vi "MGI Bezier Find k.vi"(1 "y":sgl format="%.2f", 2 "first k":i32=1, 3 "Bezier Control Points[]":sgl[](array[numeric]) format="%.2f") -> (0 "correct k":i32)   [LabVIEW 2016]
doc: "Search the Bezier Control Points array for the block containing y. y is tested against y(first k + 3 + 4*n), where n = 0, 1, .... Return value is (first k + 4*n), suitable for input to Bezier Inverse.\n\nAuthored by David A. Moore\nsupport@mooregoodideas.com\nwww.mooregoodideas.com\n\nCopyright (c) 2010, Moore Good Ideas, Inc.\n\nAll rights reserved.\n\nRedistribution and use in source and binary forms, with or without modification, are permitted provided that the following conditions are met:\n\n * Redistributions of source code must retain the above copyright notice, this list of conditions and the following disclaimer.\n * Redistributions in binary form must reproduce the above copyright notice, this list of conditions and the following disclaimer in the documentation and/or other materials provided with the distribution.\n * Neither the name of Moore Good Ideas, Inc. nor the names of its contributors may be used to endorse or promote products derived from this software without specific prior written permission.\n\nTHIS SOFTWARE IS PROVIDED BY THE COPYRIGHT HOLDERS AND CONTRIBUTORS \"AS IS\" AND ANY EXPRESS OR IMPLIED WARRANTIES, INCLUDING, BUT NOT LIMITED TO, THE IMPLIED WARRANTIES OF MERCHANTABILITY AND FITNESS FOR A PARTICULAR PURPOSE ARE DISCLAIMED. IN NO EVENT SHALL THE COPYRIGHT OWNER OR CONTRIBUTORS BE LIABLE FOR ANY DIRECT, INDIRECT, INCIDENTAL, SPECIAL, EXEMPLARY, OR CONSEQUENTIAL DAMAGES (INCLUDING, BUT NOT LIMITED TO, PROCUREMENT OF SUBSTITUTE GOODS OR SERVICES; LOSS OF USE, DATA, OR PROFITS; OR BUSINESS INTERRUPTION) HOWEVER CAUSED AND ON ANY THEORY OF LIABILITY, WHETHER IN CONTRACT, STRICT LIABILITY, OR TORT (INCLUDING NEGLIGENCE OR OTHERWISE) ARISING IN ANY WAY OUT OF THE USE OF THIS SOFTWARE, EVEN IF ADVISED OF THE POSSIBILITY OF SUCH DAMAGE."
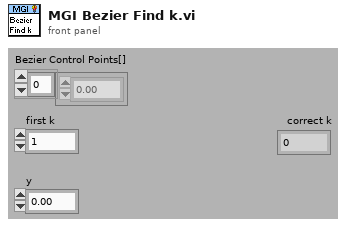
[diagram p1: front panel]
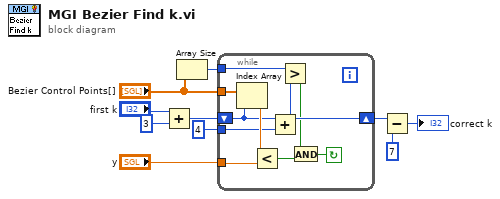
[diagram p0: block diagram]
diagram:
  n1 = Add(x="first k", y=3) -> (x+y=w1:i32)
  n2 = Array Size(array="Bezier Control Points[]") -> (size(s)=w7:i32)
  n3 = while {
    tunnel: "Bezier Control Points[]" -> [w20]
    tunnel: "y" -> [w18]
    shift-right: [w15] -> w6
    shift-left: w1 -> [w11]
    tunnel: 4 -> [w17]
    tunnel: w7 -> [w16]
    stop <- w12 continue-if-true
    n4 = Index Array(array=w20, index=w11) -> (element=w19:sgl)
    n5 = Less?(x=w19, y=w18) -> (x < y?=w14:bool)
    n6 = Add(x=w11, y=w17) -> (x+y=w15:i32)
    n7 = Greater?(x=w16, y=w15) -> (0:w13:bool)
    n8 = And(x=w13, y=w14) -> (x .and. y?=w12:bool)
  }
  n9 = Subtract(x=w6, y=7) -> (x-y=→"correct k":i32)
